vi "Run Bfr Rx - CachedSize - Check Cache.vi"(8 "error in (no error)":errorcluster, 10 "Data in":u8[](array[numeric]), 11 "Cached Buffer in":T1 {"Cache Buffer" format="%016x"}) -> (0 "error out":errorcluster, 2 "Data out":u8[](array[numeric]), 3 "Cached Buffer out":T1 {"Cache Buffer" format="%016x"}, 4 "Copy and Flush":bool, 6 "Data Size out":u64)   [LabVIEW 2016, in "UDP-Custom-Device Engine.lvlib"]
uses:
  UDP-Custom-Device Engine.lvlib
  Types/Engine - Buffered Rx Cached Buffer.ctl
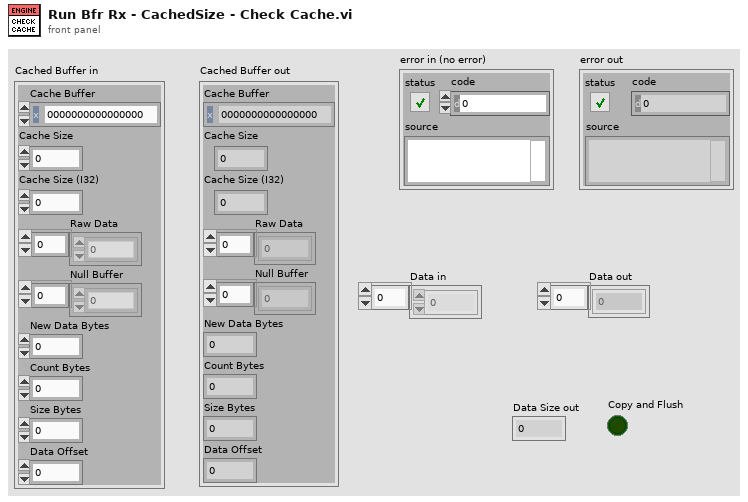
[diagram p1: front panel]
types:
  T1 = typedef "UDP-Custom-Device Engine.lvlib/Engine - Buffered Rx Cached Buffer.ctl" = cluster{"Cache Buffer":u64, "Cache Size":u64, "Cache Size (I32)":i32, "Raw Data":u8[], "Null Buffer":u8[], "New Data Bytes":u64, "Count Bytes":u64, "Size Bytes":u64, "Data Offset":u64}
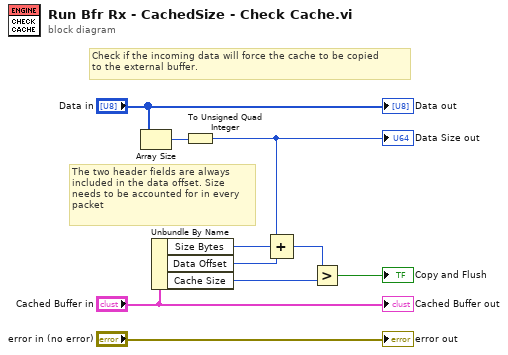
[diagram p0: block diagram]
diagram:
  # "Check if the incoming data will force the cache to be copied\nto the external buffer."
  # "The two header fields are always\nincluded in the data offset. Size\nneeds to be accounted for in every\npacket"
  n1 = Array Size(array="Data in") -> (size(s)=w6:i32)
  n2 = Unbundle By Name("Cached Buffer in") -> ("Size Bytes"=w3:u64, "Data Offset"=w4:u64, "Cache Size"=w9:u64)
  n3 = To Unsigned Quad Integer(1:w6) -> (0:w1:u64)
  "Data Size out" <- w1
  n4 = Compound Arithmetic op=ADD(w1, w3, w4) -> (w2:u64)
  n5 = Greater?(x=w2, y=w9) -> (0:→"Copy and Flush":bool)
  "error out" <- "error in (no error)"
  "Cached Buffer out" <- "Cached Buffer in"
  "Data out" <- "Data in"
